vi "Get Re from X using calibration data (array).vi"(1 "Monotonic":bool=TRUE, 2 "X []":dbl[](array[numeric]), 3 "Re cal.[]":dbl[](array[numeric]), 4 "X cal.[]":dbl[](array[numeric])) -> (0 "Re []":dbl[](array[numeric]))   [LabVIEW 2020]
doc: "Get Re = f(X) for an array of X using the calibration data as a lookup table.\n(Monotonic) cubic spline interpolation.\nPN 05-NOV-23."
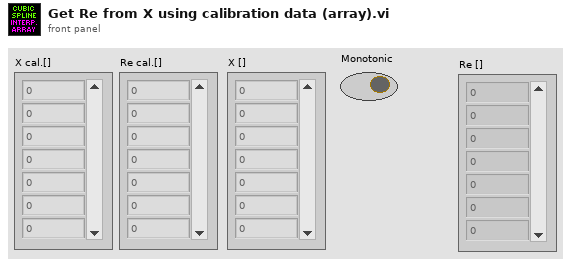
[diagram p1: front panel]
types:
  T1 = typedef "Calibration data.ctl" = cluster{"X cal.[]":dbl[], "Re cal.[]":dbl[], "a1[]":dbl[], "a2[]":dbl[], "a3[]":dbl[]}
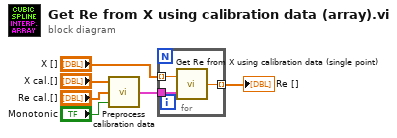
[diagram p0: block diagram]
diagram:
  n1 = call "Preprocess calibration data.vi"("Monotonic"="Monotonic", "Re cal.[]"="Re cal.[]", "X cal.[]"="X cal.[]") -> ("Calibration data"=w5:T1)
  n2 = for {
    tunnel: [w9] -> w4 mode=indexing
    tunnel: w5 -> [w8]
    tunnel: "X []" -> [w7] mode=indexing
    n3 = call "Get Re from X using calibration data (single point).vi"("Calibration data"=w8, "X"=w7) -> ("Re"=w9:dbl)
  }
  "Re []" <- w4
